vi "Validate Hardware Settings.vi"(8 "error in":errorcluster, 11 "Module Configuration in":refnum<class "Module Configuration.lvclass">) -> (0 "error out":errorcluster, 1 "Result Messages":T1[](array[typedef]), 2 "Config OK":bool, 3 "Module Configuration out":refnum<class "Module Configuration.lvclass">)   [LabVIEW 2020, in "Plugin.lvlib" / "Plugin_Controller.lvclass"]
doc: "Validate the hardware settings for test execution."
uses:
  Plugin_Controller.lvclass
  builds/Libraries/LabSys Framework.lvlibp/Configuration Storage/Module Configuration/Module Configuration.lvclass
  builds/Libraries/LabSys Framework.lvlibp/Data Node/Data Node/Result.ctl
  builds/Libraries/LabSys Framework.lvlibp/Data Node/Data Node/Result Type.ctl
  Typedefs/Connection type.ctl
  UI_Class/Plugin_UI.lvclass
  builds/Libraries/LabSys Framework.lvlibp/Data Node/Data Node/Data Node.lvclass
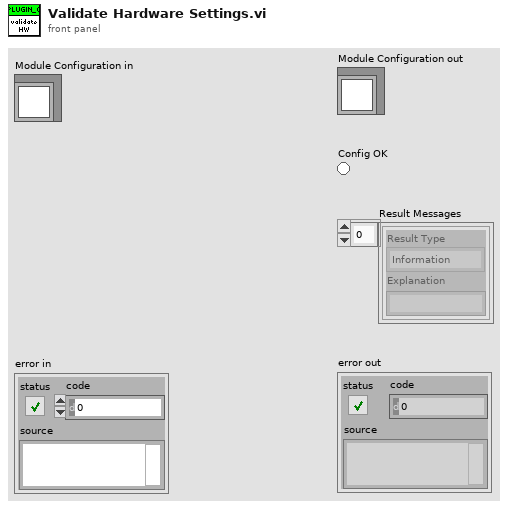
[diagram p1: front panel]
types:
  T1 = typedef "LabSys Framework.lvlibp/Data Node.lvlib/Data Node.lvclass/Result.ctl" = cluster{"Result Type":T2, "Explanation":string}
  T2 = typedef "LabSys Framework.lvlibp/Data Node.lvlib/Data Node.lvclass/Result Type.ctl" = enum16{"Information", "Warning", "Error"}
  T3 = typedef "Plugin.lvlib/Plugin_Controller.lvclass/Connection type.ctl" = enum16{"Serial", "UDP"}
  T4 = typedef "Plugin.lvlib/Plugin_UI.lvclass/Serial Configuration.ctl" = cluster{"VISA":refnum<visa-resource-name>, "Interface Type":T5, "Serial Interface":T6, "Slave Address":u8}
  T5 = typedef "Shared GUI Library.lvlibp/Interface Type.ctl" = u16
  T6 = typedef "Shared GUI Library.lvlibp/Serial Interafce.ctl" = cluster{"Baud Rate":u32, "Data Bits ":u16, "Parity":enum16{"None", "Odd", "Even"}, "Stop Bits":u16}
  T7 = typedef "Plugin.lvlib/Plugin_UI.lvclass/UDP Configuration.ctl" = cluster{"Device Port Number":u16, "Device IP":string, "Timeout":i32, "Port Number":u16}
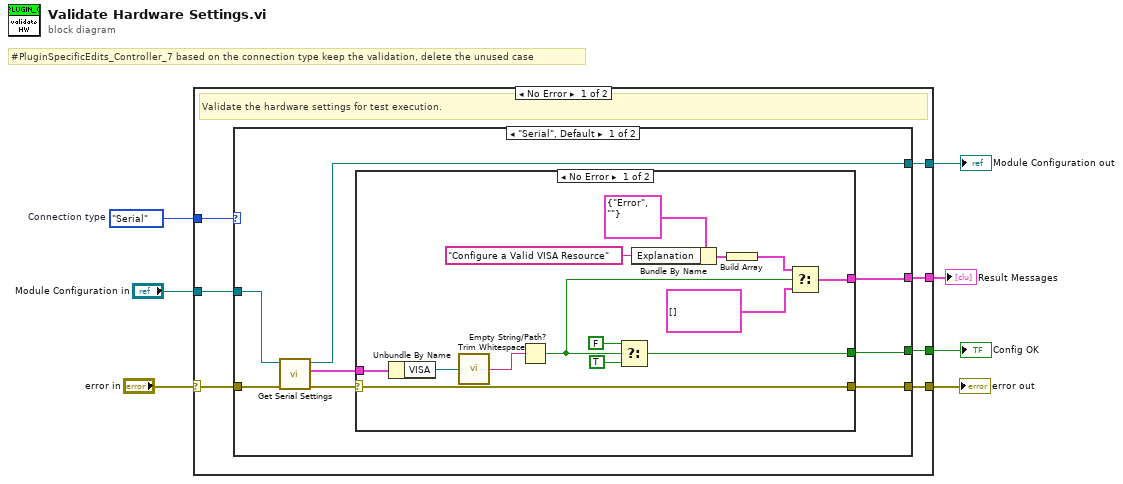
[diagram p0: block diagram]
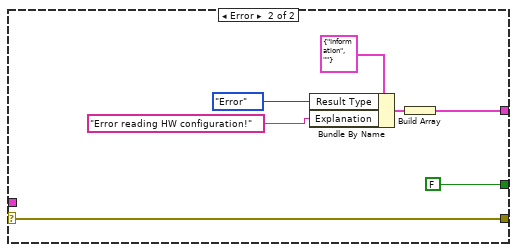
[diagram p2: hidden frame]
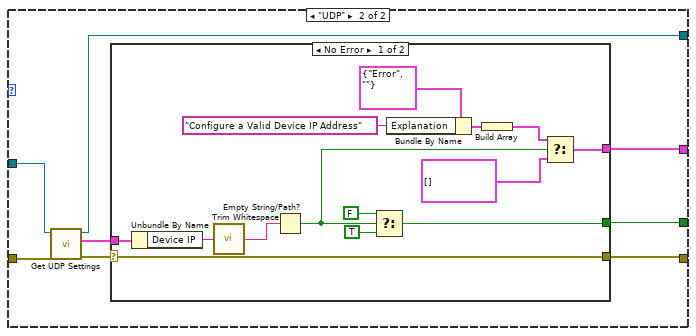
[diagram p3: hidden frame]
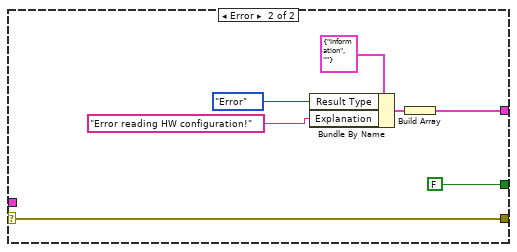
[diagram p4: hidden frame]
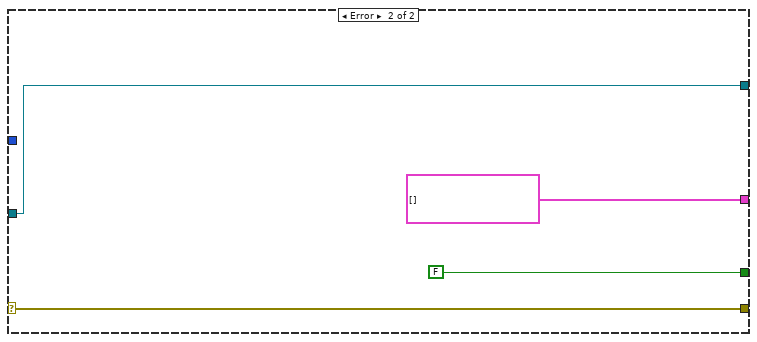
[diagram p5: hidden frame]
diagram:
  w6 = Connection_type."Serial"  # Connection type
  # "#PluginSpecificEdits_Controller_7 based on the connection type keep the validation, delete the unused case"
  n1 = case shown="No Error" "error in" {
    selector: "error in" -> [w14 w75]
    tunnel: w6 -> [w13 _]
    tunnel: "Module Configuration in" -> [w12 w76]
    tunnel: [w11 w75] -> w4
    tunnel: [w10 w76] -> w3
    tunnel: [w9 FALSE ("t")] -> w2
    tunnel: [w8 T1[] [] ("f")] -> w1
    frame No Error {
      # "Validate the hardware settings for test execution."
      n2 = case shown="\"Serial\", Default" w13 {
        tunnel: w14 -> [w22 w51]
        tunnel: w12 -> [w21 w50]
        tunnel: [w18 w46] -> w11
        tunnel: [w17 w47] -> w8
        tunnel: [w16 w45] -> w9
        tunnel: [w15 w44] -> w10
        frame "Serial", Default {
          n3 = call "Get Serial Settings.vi"("error IO"=w22, "Module Configuration in"=w21) -> ("error IO Out"=w20:errorcluster, "Serial Configuration"=w19:T4, "Module Configuration out"=w15:refnum<class "Module Configuration.lvclass">)  [unwired: 7 in]
          n4 = case shown="No Error" w20 {
            selector: w20 -> [w36 w38]
            tunnel: w19 -> [w34 _]
            tunnel: [w25 w39] -> w17
            tunnel: [w31 FALSE] -> w16
            tunnel: [w36 w38] -> w18
            frame No Error {
              n5 = Unbundle By Name(w34) -> ("VISA"=w33:refnum<visa-resource-name>)
              n6 = call <vilib>:"Trim Whitespace.vi"("string"=w33) -> ("trimmed string"=w29:string)  [unwired: 1 in]
              n7 = Empty String/Path?(string/path=w29) -> (empty?=w27:bool)
              n8 = Select(t=FALSE, s=w27, f=TRUE) -> (s? t:f=w31:bool)
              n9 = Bundle By Name(cluster=T1 {"Result Type"=enum."Error", "Explanation"=""}, "Explanation"="Configure a Valid VISA Resource") -> (w32:T1)
              n10 = Build Array(w32) -> (w26:T1[])
              n11 = Select(t=w26, s=w27, f=T1[] []) -> (s? t:f=w25:T1[])
            }
            frame Error {
              n12 = Bundle By Name(cluster=T1 {"Result Type"=enum."Information", "Explanation"=""}, "Result Type"=Result_Type."Error", "Explanation"="Error reading HW configuration!") -> (w40:T1)
              n13 = Build Array(w40) -> (w39:T1[])
            }
          }
        }
        frame "UDP" {
          n14 = call "Get UDP Settings.vi"("error in (no error)"=w51, "Module Configuration"=w50) -> ("error out"=w49:errorcluster, "UDP configuration"=w48:T7, "Module Configuration out"=w44:refnum<class "Module Configuration.lvclass">)  [unwired: 7 in]
          n15 = case shown="No Error" w49 {
            selector: w49 -> [w65 w67]
            tunnel: w48 -> [w63 _]
            tunnel: [w54 w68] -> w47
            tunnel: [w60 FALSE] -> w45
            tunnel: [w65 w67] -> w46
            frame No Error {
              n16 = Unbundle By Name(w63) -> ("Device IP"=w62:string)
              n17 = call <vilib>:"Trim Whitespace.vi"("string"=w62) -> ("trimmed string"=w58:string)  [unwired: 1 in]
              n18 = Empty String/Path?(string/path=w58) -> (empty?=w56:bool)
              n19 = Select(t=FALSE, s=w56, f=TRUE) -> (s? t:f=w60:bool)
              n20 = Bundle By Name(cluster=T1 {"Result Type"=enum."Error", "Explanation"=""}, "Explanation"="Configure a Valid Device IP Address") -> (w61:T1)
              n21 = Build Array(w61) -> (w55:T1[])
              n22 = Select(t=w55, s=w56, f=T1[] []) -> (s? t:f=w54:T1[])
            }
            frame Error {
              n23 = Bundle By Name(cluster=T1 {"Result Type"=enum."Information", "Explanation"=""}, "Result Type"=Result_Type."Error", "Explanation"="Error reading HW configuration!") -> (w69:T1)
              n24 = Build Array(w69) -> (w68:T1[])
            }
          }
        }
      }
    }
    frame Error {
    }
  }
  "error out" <- w4
  "Module Configuration out" <- w3
  "Config OK" <- w2
  "Result Messages" <- w1
